vi "Update.vi"(8 "error in (no error)":errorcluster, 10 "Message in":refnum<class "UpdateMessage.lvclass">, 11 "DAQMH121119OrcaFlash in":refnum<class "DAQOrcaFlash.lvclass">) -> (0 "error out":errorcluster, 3 "DAQMH121119OrcaFlash out":refnum<class "DAQOrcaFlash.lvclass">)   [LabVIEW 2012, in "DAQOrcaFlash.lvclass"]
doc: "The update method processes the command 'update'. \n\nThe command 'update' is used for receiving new values to be set to the private data of the class. This could be seen as a public set method for setting new parameters to the private class data."
uses:
  DAQOrcaFlash.lvclass
  <vilib>/Distrio/Murmex/UpdateMessage/UpdateMessage.lvclass
  DAQOrcaFlash.lvclass/DAQOrcaFlash.ctl
  visualisation_line_cluster.ctl
  <vilib>/Distrio/Murmex/Murmex/Murmex.lvclass
panel:
  # "This method is called when the UPDATE\ntrigger is sent. \n\nOverride this method when your component needs to\nrespond to this trigger. \n\nCall parent for proper implementation"
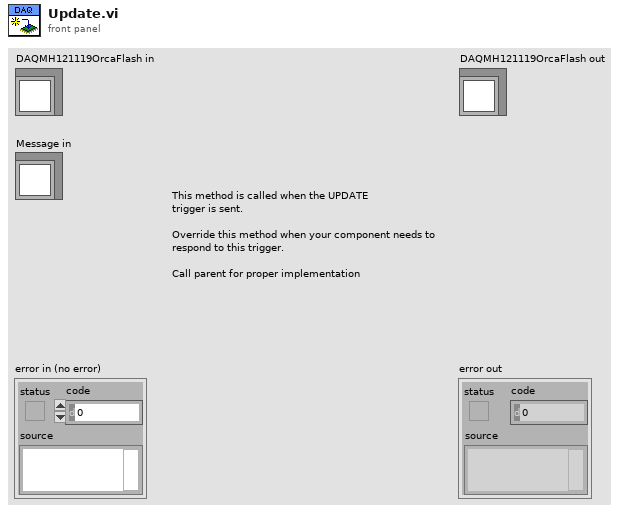
[diagram p1: front panel]
types:
  T1 = typedef "DAQOrcaFlash.lvclass/visualisation_line_cluster.ctl" = cluster{"direction":enum16{"horizontal", "vertical"}, "position":i32}
  T2 = typedef "IMAQ Image.ctl" = refnum<image>
  T3 = cluster{"Conversion Method":u32, "Minimum Value":i32, "Maximum Value":i32, "# Shifts":i32}
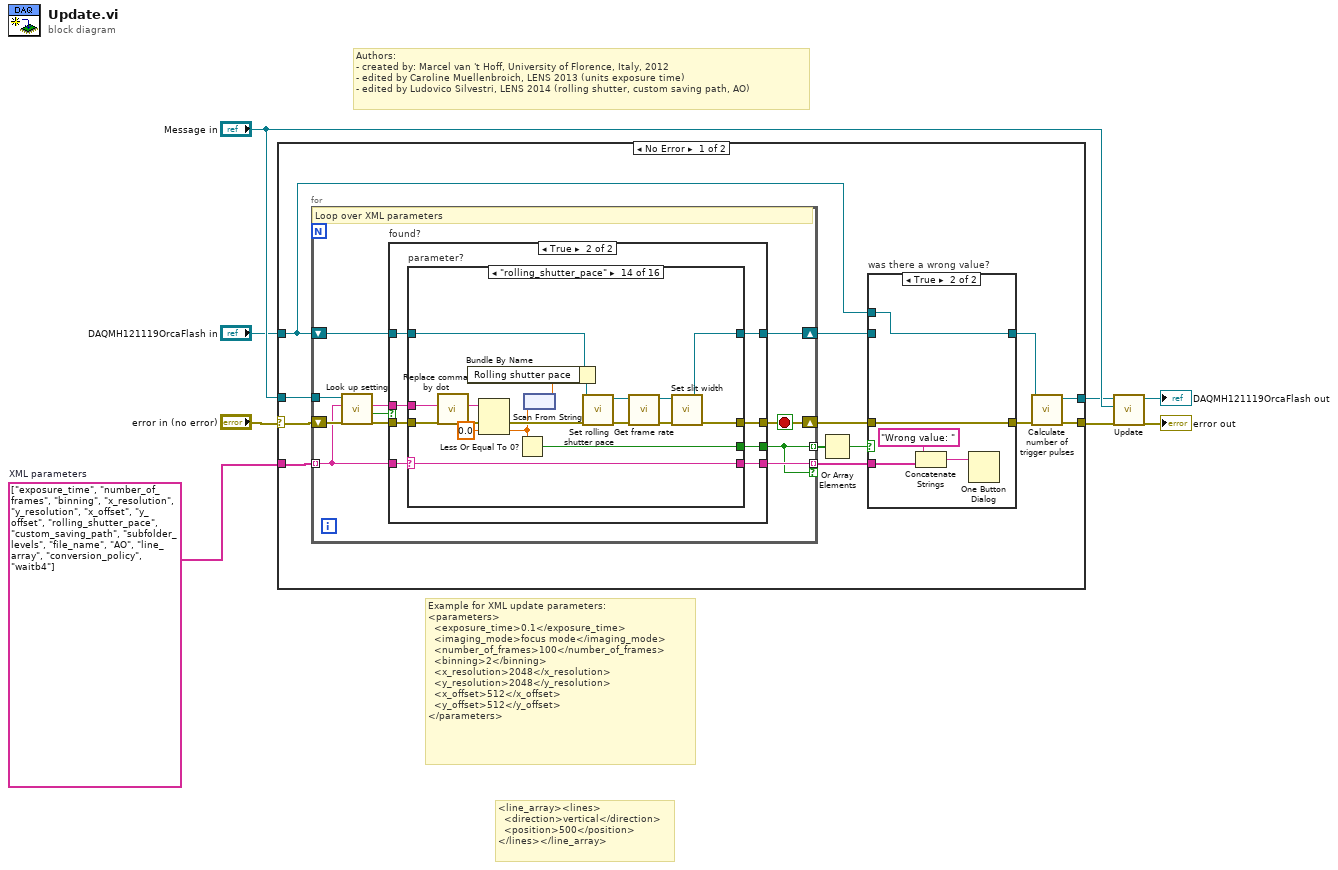
[diagram p0: block diagram]
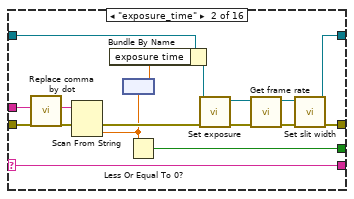
[diagram p5: hidden frame]
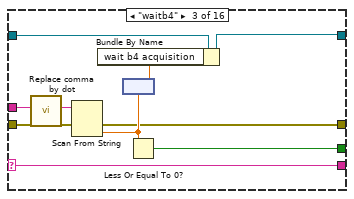
[diagram p6: hidden frame]
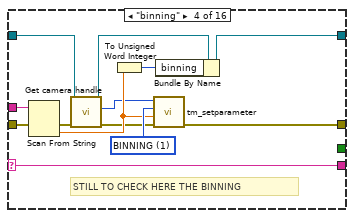
[diagram p7: hidden frame]
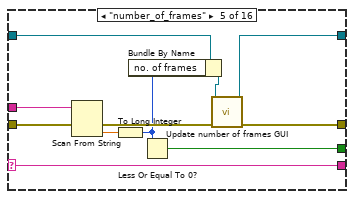
[diagram p8: hidden frame]
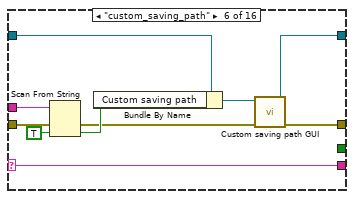
[diagram p9: hidden frame]
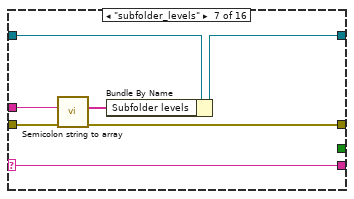
[diagram p10: hidden frame]
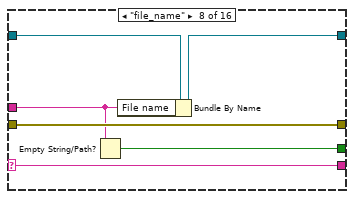
[diagram p11: hidden frame]
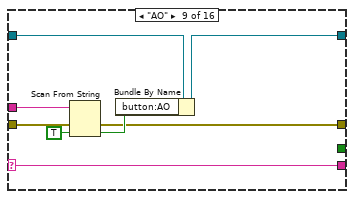
[diagram p12: hidden frame]
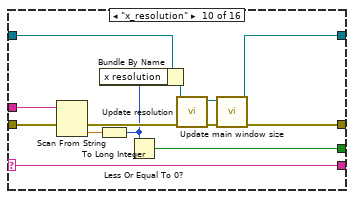
[diagram p13: hidden frame]
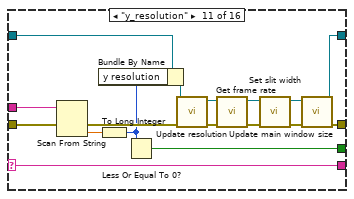
[diagram p14: hidden frame]
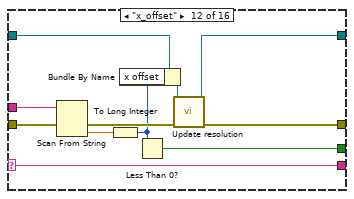
[diagram p15: hidden frame]
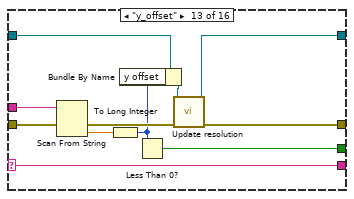
[diagram p16: hidden frame]
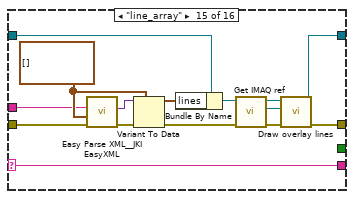
[diagram p17: hidden frame]
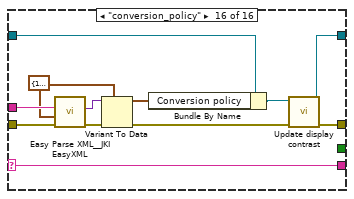
[diagram p18: hidden frame]
diagram:
  w8 = string[] ["exposure_time", "number_of_frames", "binning", "x_resolution", "y_resolution", "x_offset", "y_offset", "rolling_shutter_pace", "custom_saving_path", "subfolder_levels", "file_name", "AO", "line_array", "conversion_policy", "waitb4"]  # XML parameters
  # "<line_array><lines>\n  <direction>vertical</direction>\n  <position>500</position>\n</lines></line_array>"
  # "Example for XML update parameters:\n<parameters>\n  <exposure_time>0.1</exposure_time>\n  <imaging_mode>focus mode</imaging_mode>\n  <number_of_frames>100</number_of_frames>\n  <binning>2</binning>\n  <x_resolution>2048</x_resolution>\n  <y_resolution>2048</y_resolution>\n  <x_offset>512</x_offset>\n  <y_offset>512</y_offset>\n</parameters>"
  # "Authors: \n- created by: Marcel van 't Hoff, University of Florence, Italy, 2012\n- edited by Caroline Muellenbroich, LENS 2013 (units exposure time)\n- edited by Ludovico Silvestri, LENS 2014 (rolling shutter, custom saving path, AO)"
  n1 = case shown="No Error" "error in (no error)" {
    selector: "error in (no error)" -> [w21 w232]
    tunnel: [w18 w232] -> w3
    tunnel: [w17 w231] -> w4
    tunnel: "DAQMH121119OrcaFlash in" -> [w14 w231]
    tunnel: "Message in" -> [w20 _]
    tunnel: w8 -> [w19 _]
    frame No Error {
      n2 = for "loop over parameters" {
        shift-right: [w37] -> w9
        shift-left: w21 -> [w35]
        shift-right: [w38] -> w12
        shift-left: w14 -> [w39]
        tunnel: w20 -> [w36]
        tunnel: w19 -> [w33] mode=indexing
        tunnel: [w29] -> w16 mode=indexing
        tunnel: [w30] -> w11 mode=indexing if=w29
        stop <- w37 stop-if-true
        # "Loop over XML parameters"
        n3 = call <vilib>:"Look up setting.vi"("error in (no error)"=w35, "tag name"=w33, "UpdateMessage in"=w36) -> ("error out"=w34:errorcluster, "found?"=w32:bool, "value"=w31:string)  [unwired: 5 in, 1 out]
        n4 = case "found?" shown="True" w32 {
          tunnel: w34 -> [w41 w50]
          tunnel: w31 -> [_ w49]
          tunnel: w33 -> [w40 w48]
          tunnel: w39 -> [w42 w47]
          tunnel: [w41 w46] -> w37
          tunnel: [w42 w45] -> w38
          tunnel: [_ w44] -> w29
          tunnel: [w40 w43] -> w30
          frame False {
          }
          frame True {
            # "XML parameter found?"
            n5 = case "parameter?" shown="\"rolling_shutter_pace\"" w48 {
              selector: w48 -> [w51 w54 w72 w80 w95 w104 w114 w123 w127 w135 w148 w165 w176 w187 w204 w219]
              tunnel: w50 -> [w52 w69 w79 w92 w102 w110 w118 w124 w133 w145 w162 w173 w184 w202 w214 w227]
              tunnel: w49 -> [_ w68 w78 w91 w101 w111 w116 w122 w132 w146 w163 w174 w185 w192 w215 w228]
              tunnel: w47 -> [w53 w59 w75 w84 w103 w113 w120 w126 w131 w147 w164 w175 w186 w203 w213 w226]
              tunnel: [w52 w63 w71 w86 w98 w107 w117 w124 w128 w141 w151 w169 w181 w197 w206 w223] -> w46
              tunnel: [w53 w62 w70 w90 w96 w105 w119 w125 w129 w139 w153 w168 w179 w196 w208 w222] -> w45
              tunnel: [_ w55 w73 _ w93 _ _ w121 _ w136 w149 w166 w177 w188 _ _] -> w44
              tunnel: [w51 w54 w72 w80 w95 w104 w114 w123 w127 w135 w148 w165 w176 w187 w204 w219] -> w43
              frame Default {
              }
              frame "exposure_time" {
                n6 = call <vilib>:"Replace comma by dot.vi"("input string"=w68) -> ("result string"=w66:string)  [unwired: 10 in]
                n7 = Scan From String(input string=w66, error in=w69) -> (error out=w57:errorcluster, output 1=w56:dbl)  [unwired: 3 in, 2 out]
                n8 = node(w56) -> (w67:dbl[unit])
                n9 = Bundle By Name(cluster=w59, "exposure time"=w67) -> (w58:refnum<class "DAQOrcaFlash.lvclass">)
                n10 = Less Or Equal To 0?(x=w56) -> (x <= 0?=w55:bool)
                n11 = call-dynamic "Set exposure.vi"("error in (no error)"=w57, "DAQOrcaFlash in"=w58) -> ("error out"=w61:errorcluster, "DAQOrcaFlash out"=w60:refnum<class "DAQOrcaFlash.lvclass">)  [unwired: 8 in]
                n12 = call-dynamic "Get frame rate.vi"("error in (no error)"=w61, "DAQOrcaFlash in"=w60) -> ("error out"=w64:errorcluster, "DAQOrcaFlash out"=w65:refnum<class "DAQOrcaFlash.lvclass">)  [unwired: 8 in]
                n13 = call-dynamic "Set slit width.vi"("error in (no error)"=w64, "DAQOrcaFlash in"=w65) -> ("error out"=w63:errorcluster, "DAQOrcaFlash out"=w62:refnum<class "DAQOrcaFlash.lvclass">)  [unwired: 8 in]
              }
              frame "waitb4" {
                n14 = call <vilib>:"Replace comma by dot.vi"("input string"=w78) -> ("result string"=w76:string)  [unwired: 10 in]
                n15 = Scan From String(input string=w76, error in=w79) -> (error out=w71:errorcluster, output 1=w74:dbl)  [unwired: 3 in, 2 out]
                n16 = node(w74) -> (w77:dbl[unit])
                n17 = Bundle By Name(cluster=w75, "wait b4 acquisition"=w77) -> (w70:refnum<class "DAQOrcaFlash.lvclass">)
                n18 = Less Or Equal To 0?(x=w74) -> (x <= 0?=w73:bool)
              }
              frame "binning" {
                w89 = 1 items=["BINNING"=1, "BITS PER CHANNEL"=2, "ACTIVE VIEW INDEX"=3, "CCD MODE"=4, "SENSOR MODE"=5, "READOUT MODE"=6, "EXPOSURE TIME"=7, "CONTRAST GAIN"=8, "CONTRAST OFFSET"=9, "LIGHT MODE"=10, "SENSITIVITY"=11, "WHITE BALANCE"=12, "PHOTON IMAGING MODE"=13, "HIGH DYNAMIC RANGE MODE"=14, "TRIGGER SOURCE"=15, "TRIGGER ACTIVE"=16, "TRIGGER MODE"=17, "TRIGGER POLARITY"=18, "TRIGGER GLOBAL EXPOSURE"=19, "FIRST TRIGGER BEHAVIOR"=20, "TRIGGER TIMES"=21, "OUTPUT TRIGGER POLARITY"=22, "OUTPUT TRIGGER DELAY"=23, "OUTPUT TRIGGER PERIOD"=24, "TEMPERATURE"=25, "TEMPERATURE TARGET"=26, "SENSOR COOLER FAN"=27, "MECHANICAL SHUTTER"=28, "BACK FOCUS POSITION"=29, "FRAMEBUNDLE MODE"=30, "FRAMEBUNDLE NUMBER"=31] ("Parameter")
                # "STILL TO CHECK HERE THE BINNING"
                n19 = Scan From String(input string=w91, error in=w92) -> (error out=w87:errorcluster, output 1=w88:dbl)  [unwired: 3 in, 2 out]
                n20 = call "Get camera handle.vi"("error in (no error)"=w87, "DAQMH121119OrcaFlash in"=w84) -> ("error out"=w85:errorcluster, "cam handle"=w82:u32, "DAQMH121119OrcaFlash out"=w83:refnum<class "DAQOrcaFlash.lvclass">)  [unwired: 7 in]
                n21 = To Unsigned Word Integer(number=w88) -> (unsigned 16bit integer=w81:u16)
                n22 = call <userlib>:"tm_setparameter.vi"("error in (no error)"=w85, "Value in"=w88, "Parameter"=w89, "Handle in"=w82) -> ("error out"=w86:errorcluster)  [unwired: 6 in, 1 out]
                n23 = Bundle By Name(cluster=w83, "binning"=w81) -> (w90:refnum<class "DAQOrcaFlash.lvclass">)
              }
              frame "number_of_frames" {
                n24 = Scan From String(input string=w101, error in=w102) -> (error out=w99:errorcluster, output 1=w100:dbl)  [unwired: 3 in, 2 out]
                n25 = To Long Integer(number=w100) -> (32bit integer=w94:i32)
                n26 = Bundle By Name(cluster=w103, "no. of frames"=w94) -> (w97:refnum<class "DAQOrcaFlash.lvclass">)
                n27 = Less Or Equal To 0?(x=w94) -> (x <= 0?=w93:bool)
                n28 = call-dynamic "Update number of frames GUI.vi"("error in (no error)"=w99, "DAQOrcaFlash in"=w97) -> ("error out"=w98:errorcluster, "DAQOrcaFlash out"=w96:refnum<class "DAQOrcaFlash.lvclass">)  [unwired: 8 in]
              }
              frame "custom_saving_path" {
                n29 = Scan From String(input string=w111, error in=w110, default 1=TRUE) -> (error out=w108:errorcluster, output 1=w109:bool)  [unwired: 2 in, 2 out]
                n30 = Bundle By Name(cluster=w113, "Custom saving path"=w109) -> (w106:refnum<class "DAQOrcaFlash.lvclass">)
                n31 = call-dynamic "Custom saving path GUI.vi"("error in (no error)"=w108, "DAQOrcaFlash in"=w106) -> ("error out"=w107:errorcluster, "DAQOrcaFlash out"=w105:refnum<class "DAQOrcaFlash.lvclass">)  [unwired: 8 in]
              }
              frame "subfolder_levels" {
                n32 = call "Semicolon string to array.vi"("error in"=w118, "Semicolon string"=w116) -> ("error out"=w117:errorcluster, "String array"=w115:string[])  [unwired: 8 in]
                n33 = Bundle By Name(cluster=w120, "Subfolder levels"=w115) -> (w119:refnum<class "DAQOrcaFlash.lvclass">)
              }
              frame "file_name" {
                n34 = Empty String/Path?(string/path=w122) -> (empty?=w121:bool)
                n35 = Bundle By Name(cluster=w126, "File name"=w122) -> (w125:refnum<class "DAQOrcaFlash.lvclass">)
              }
              frame "AO" {
                n36 = Scan From String(input string=w132, error in=w133, default 1=TRUE) -> (error out=w128:errorcluster, output 1=w130:bool)  [unwired: 2 in, 2 out]
                n37 = Bundle By Name(cluster=w131, "button:AO"=w130) -> (w129:refnum<class "DAQOrcaFlash.lvclass">)
              }
              frame "x_resolution" {
                n38 = Scan From String(input string=w146, error in=w145) -> (error out=w138:errorcluster, output 1=w144:dbl)  [unwired: 3 in, 2 out]
                n39 = To Long Integer(number=w144) -> (32bit integer=w137:i32)
                n40 = Bundle By Name(cluster=w147, "x resolution"=w137) -> (w143:refnum<class "DAQOrcaFlash.lvclass">)
                n41 = Less Or Equal To 0?(x=w137) -> (x <= 0?=w136:bool)
                n42 = call "Update resolution.vi"("error in (no error)"=w138, "DAQMH121119OrcaFlash in"=w143) -> ("error out"=w142:errorcluster, "DAQMH121119OrcaFlash out"=w140:refnum<class "DAQOrcaFlash.lvclass">)  [unwired: 8 in]
                n43 = call "Update main window size.vi"("error in (no error)"=w142, "DAQOrcaFlash in"=w140) -> ("error out"=w141:errorcluster, "DAQOrcaFlash out"=w139:refnum<class "DAQOrcaFlash.lvclass">)  [unwired: 8 in]
              }
              frame "y_resolution" {
                n44 = Scan From String(input string=w163, error in=w162) -> (error out=w160:errorcluster, output 1=w161:dbl)  [unwired: 3 in, 2 out]
                n45 = To Long Integer(number=w161) -> (32bit integer=w150:i32)
                n46 = Bundle By Name(cluster=w164, "y resolution"=w150) -> (w159:refnum<class "DAQOrcaFlash.lvclass">)
                n47 = Less Or Equal To 0?(x=w150) -> (x <= 0?=w149:bool)
                n48 = call "Update resolution.vi"("error in (no error)"=w160, "DAQMH121119OrcaFlash in"=w159) -> ("error out"=w156:errorcluster, "DAQMH121119OrcaFlash out"=w155:refnum<class "DAQOrcaFlash.lvclass">)  [unwired: 8 in]
                n49 = call-dynamic "Get frame rate.vi"("error in (no error)"=w156, "DAQOrcaFlash in"=w155) -> ("error out"=w158:errorcluster, "DAQOrcaFlash out"=w157:refnum<class "DAQOrcaFlash.lvclass">)  [unwired: 8 in]
                n50 = call-dynamic "Set slit width.vi"("error in (no error)"=w158, "DAQOrcaFlash in"=w157) -> ("error out"=w152:errorcluster, "DAQOrcaFlash out"=w154:refnum<class "DAQOrcaFlash.lvclass">)  [unwired: 8 in]
                n51 = call "Update main window size.vi"("error in (no error)"=w152, "DAQOrcaFlash in"=w154) -> ("error out"=w151:errorcluster, "DAQOrcaFlash out"=w153:refnum<class "DAQOrcaFlash.lvclass">)  [unwired: 8 in]
              }
              frame "x_offset" {
                n52 = Scan From String(input string=w174, error in=w173) -> (error out=w171:errorcluster, output 1=w172:dbl)  [unwired: 3 in, 2 out]
                n53 = To Long Integer(number=w172) -> (32bit integer=w167:i32)
                n54 = Bundle By Name(cluster=w175, "x offset"=w167) -> (w170:refnum<class "DAQOrcaFlash.lvclass">)
                n55 = Less Than 0?(x=w167) -> (x < 0?=w166:bool)
                n56 = call "Update resolution.vi"("error in (no error)"=w171, "DAQMH121119OrcaFlash in"=w170) -> ("error out"=w169:errorcluster, "DAQMH121119OrcaFlash out"=w168:refnum<class "DAQOrcaFlash.lvclass">)  [unwired: 8 in]
              }
              frame "y_offset" {
                n57 = Scan From String(input string=w185, error in=w184) -> (error out=w182:errorcluster, output 1=w183:dbl)  [unwired: 3 in, 2 out]
                n58 = To Long Integer(number=w183) -> (32bit integer=w178:i32)
                n59 = Bundle By Name(cluster=w186, "y offset"=w178) -> (w180:refnum<class "DAQOrcaFlash.lvclass">)
                n60 = Less Than 0?(x=w178) -> (x < 0?=w177:bool)
                n61 = call "Update resolution.vi"("error in (no error)"=w182, "DAQMH121119OrcaFlash in"=w180) -> ("error out"=w181:errorcluster, "DAQMH121119OrcaFlash out"=w179:refnum<class "DAQOrcaFlash.lvclass">)  [unwired: 8 in]
              }
              frame "rolling_shutter_pace" {
                n62 = call <vilib>:"Replace comma by dot.vi"("input string"=w192) -> ("result string"=w191:string)  [unwired: 10 in]
                n63 = Scan From String(input string=w191, error in=w202, default 1=sgl 0.0 ("default value 1")) -> (error out=w201:errorcluster, output 1=w189:sgl)  [unwired: 2 in, 2 out]
                n64 = Less Or Equal To 0?(x=w189) -> (x <= 0?=w188:bool)
                n65 = node(w189) -> (w190:sgl[unit])
                n66 = Bundle By Name(cluster=w203, "Rolling shutter pace"=w190) -> (w200:refnum<class "DAQOrcaFlash.lvclass">)
                n67 = call-dynamic "Set rolling shutter pace.vi"("error in (no error)"=w201, "DAQOrcaFlash in"=w200) -> ("error out"=w199:errorcluster, "DAQOrcaFlash out"=w195:refnum<class "DAQOrcaFlash.lvclass">)  [unwired: 8 in]
                n68 = call-dynamic "Get frame rate.vi"("error in (no error)"=w199, "DAQOrcaFlash in"=w195) -> ("error out"=w198:errorcluster, "DAQOrcaFlash out"=w194:refnum<class "DAQOrcaFlash.lvclass">)  [unwired: 8 in]
                n69 = call-dynamic "Set slit width.vi"("error in (no error)"=w198, "DAQOrcaFlash in"=w194) -> ("error out"=w197:errorcluster, "DAQOrcaFlash out"=w196:refnum<class "DAQOrcaFlash.lvclass">)  [unwired: 8 in]
              }
              frame "line_array" {
                w217 = T1[] [] ("lines")
                n70 = call <vilib>:"Easy Parse XML__JKI EasyXML.vi"("error in (no error)"=w214, "LabVIEW Data (Type)"=w217, "XML String"=w215) -> ("error out"=w218:errorcluster, "LabVIEW Data"=w216:variant)  [unwired: 7 in]
                n71 = Variant To Data(error in=w218, type=w217, Variant=w216) -> (data=w212:T1[], error out=w211:errorcluster)
                n72 = Bundle By Name(cluster=w213, "lines"=w212) -> (w209:refnum<class "DAQOrcaFlash.lvclass">)
                n73 = call "Get IMAQ ref.vi"("error in (no error)"=w211, "DAQMH121119OrcaFlash in"=w209) -> ("error out"=w207:errorcluster, "IMAQ reference"=w205:T2, "DAQMH121119OrcaFlash out"=w210:refnum<class "DAQOrcaFlash.lvclass">)  [unwired: 7 in]
                n74 = call "Draw overlay lines.vi"("error in (no error)"=w207, "IMAQ reference"=w205, "DAQOrcaFlash in"=w210) -> ("error out"=w206:errorcluster, "DAQOrcaFlash out"=w208:refnum<class "DAQOrcaFlash.lvclass">)  [unwired: 6 in, 1 out]
              }
              frame "conversion_policy" {
                w220 = T3 {"Conversion Method"=10, "Minimum Value"=0, "Maximum Value"=1000, "# Shifts"=0} ("Conversion policy")
                n75 = call <vilib>:"Easy Parse XML__JKI EasyXML.vi"("error in (no error)"=w227, "LabVIEW Data (Type)"=w220, "XML String"=w228) -> ("error out"=w230:errorcluster, "LabVIEW Data"=w229:variant)  [unwired: 7 in]
                n76 = Variant To Data(error in=w230, type=w220, Variant=w229) -> (data=w225:T3, error out=w224:errorcluster)
                n77 = Bundle By Name(cluster=w226, "Conversion policy"=w225) -> (w221:refnum<class "DAQOrcaFlash.lvclass">)
                n78 = call-dynamic "Update display contrast.vi"("error in (no error)"=w224, "DAQOrcaFlash in"=w221) -> ("error out"=w223:errorcluster, "DAQOrcaFlash out"=w222:refnum<class "DAQOrcaFlash.lvclass">)  [unwired: 8 in]
              }
            }
          }
        }
      }
      n79 = Or Array Elements(Boolean array=w16) -> (logical OR=w15:bool)
      n80 = case "was there a wrong value?" shown="True" w15 {
        tunnel: w14 -> [_ w28]
        tunnel: [w23 w28] -> w13
        tunnel: w12 -> [w23 _]
        tunnel: w11 -> [_ w27]
        tunnel: [w22 w24] -> w10
        tunnel: w9 -> [w22 w24]
        frame False {
        }
        frame True {
          n81 = Concatenate Strings("Wrong value: " ("message"), w27) -> (w25:string)
          n82 = One Button Dialog(message=w25) -> ()  [unwired: 1 in, 1 out]
        }
      }
      n83 = call "Calculate number of trigger pulses.vi"("error in (no error)"=w10, "DAQOrcaFlash in"=w13) -> ("error out"=w18:errorcluster, "DAQOrcaFlash out"=w17:refnum<class "DAQOrcaFlash.lvclass">)  [unwired: 8 in]
    }
    frame Error {
    }
  }
  n84 = call-parent "Update.vi"("error in (no error)"=w3, "Message in"="Message in", "Murmex in"=w4) -> ("error out"=→"error out":errorcluster, "Murmex out"=→"DAQMH121119OrcaFlash out":refnum<class "DAQOrcaFlash.lvclass">)  [unwired: 7 in]
